vi "Download Log Files.vi"(7 "Target Directory (\"\": Use Temporary Dir)":path, 8 "error in (no error)":errorcluster, 9 "Log Files to Download":path[](array[path]), 10 "Session Name in":string, 11 "Data Logging Manager Ref in":T1) -> (0 "error out":errorcluster, 1 "Resolved Log File Paths":path[](array[path]), 2 "Session Name out":string, 3 "Data Logging Manager Ref out":T1, 4 "Log File Download Errors":errorcluster[](array[cluster]))   [LabVIEW 2020, in "NI_VS Data Logging API.lvlib"]
uses:
  <vilib>/NI VeriStand/Execution/DataLogging/NI_VS Data Logging API.lvlib
  <vilib>/NI VeriStand/Execution/DataLogging/IDataLogging Ref.ctl
  NationalInstruments.VeriStand.ClientAPI
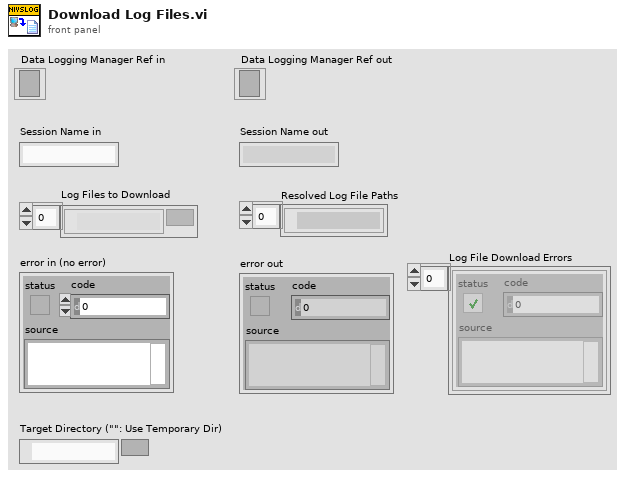
[diagram p1: front panel]
types:
  T1 = typedef "NI_VS Data Logging API.lvlib/IDataLogging Ref.ctl" = refnum<k24>
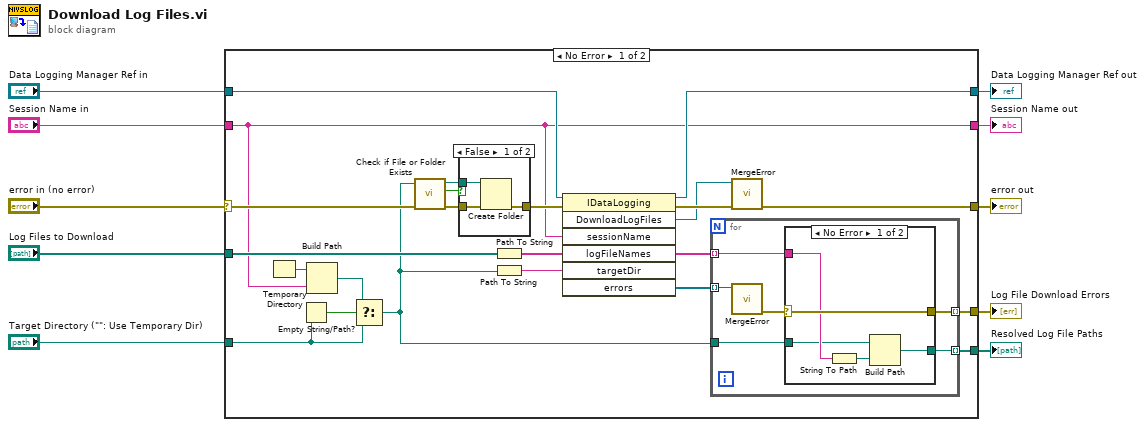
[diagram p0: block diagram]
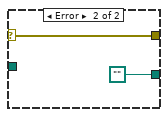
[diagram p3: hidden frame]
diagram:
  n1 = case shown="No Error" "error in (no error)" {
    selector: "error in (no error)" -> [w26 w53]
    tunnel: "Data Logging Manager Ref in" -> [w32 w52]
    tunnel: [w31 w52] -> w9
    tunnel: [w30 w53] -> w7
    tunnel: "Session Name in" -> [w12 w51]
    tunnel: "Log Files to Download" -> [w29 _]
    tunnel: "Target Directory (\"\": Use Temporary Dir)" -> [w18 _]
    tunnel: [w28 _] -> w3
    tunnel: [w12 w51] -> w2
    tunnel: [w27 _] -> w1
    frame No Error {
      n2 = Temporary Directory() -> (w13:path)
      n3 = Empty String/Path?(string/path=w18) -> (empty?=w19:bool)
      n4 = Build Path(base path=w13, name or relative path=w12) -> (appended path=w11:path)
      n5 = Select(t=w11, s=w19, f=w18) -> (s? t:f=w17:path)
      n6 = call <vilib>:"Check if File or Folder Exists.vi"("error in (no error)"=w26, "path"=w17) -> ("error out"=w16:errorcluster, "file or folder exists?"=w15:bool, "dup path"=w14:path)  [unwired: 7 in]
      n7 = case shown="False" w15 {
        tunnel: w16 -> [w36 w37]
        tunnel: [w34 w37] -> w33
        tunnel: w14 -> [w35 _]
        frame False {
          n8 = Create Folder(path (use dialog)=w35, error in=w36) -> (error out=w34:errorcluster)  [unwired: 1 in, 2 out]
        }
        frame True {
        }
      }
      n9 = Path To String(path=w29) -> (string=w23:string[])
      n10 = Path To String(path=w17) -> (string=w22:string)
      n11 = invoke class="IDataLogging" method="DownloadLogFiles"(reference=w32, error in=w33, "sessionName"=w12, "logFileNames"=w23, "targetDir"=w22) -> (reference out=w31:T1, error out=w25:errorcluster, "DownloadLogFiles"=w24:refnum<k24>, "logFileNames"=w20:string[], "errors"=w21:refnum<k24>[])  [unwired: 2 in, 2 out]
      n12 = for {
        tunnel: w21 -> [w43] mode=indexing
        tunnel: [w41] -> w28 mode=indexing
        tunnel: w20 -> [w40] mode=indexing
        tunnel: w17 -> [w39]
        tunnel: [w38] -> w27 mode=indexing
        n13 = call <vilib>:"MergeError.vi"("Error"=w43) -> ("error out"=w42:errorcluster)  [unwired: 10 in]
        n14 = case shown="No Error" w42 {
          selector: w42 -> [w48 w49]
          tunnel: [w48 w49] -> w41
          tunnel: w40 -> [w47 _]
          tunnel: w39 -> [w45 _]
          tunnel: [w44 path ""] -> w38
          frame No Error {
            n15 = String To Path(string=w47) -> (path=w46:path)
            n16 = Build Path(base path=w45, name or relative path=w46) -> (appended path=w44:path)
          }
          frame Error {
          }
        }
      }
      n17 = call <vilib>:"MergeError.vi"("error in (no error)"=w25, "Error"=w24) -> ("error out"=w30:errorcluster)  [unwired: 9 in]
    }
    frame Error {
    }
  }
  "Data Logging Manager Ref out" <- w9
  "error out" <- w7
  "Session Name out" <- w2
  "Log File Download Errors" <- w3
  "Resolved Log File Paths" <- w1
